vi "tcp client test.vi"() -> ()   [LabVIEW 2015]
panel:
  in  "FUNC":bool
  in  "test":bool=TRUE
  in  "string":string="stastic"
  in  "Direct program":T1
  in  "Boolean":bool
  out "error constant 2":errorcluster
  in  "data":string
  in  "stop":bool
  out "remote address":string
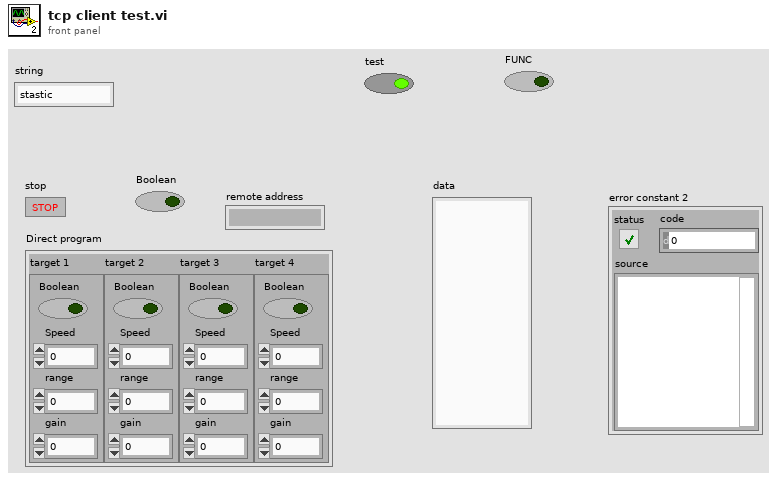
[diagram p1: front panel]
types:
  T1 = cluster{"target 1":cluster{"Boolean":bool, "Speed":dbl, "range":dbl, "gain":dbl}, "target 2":cluster{"Boolean":bool, "Speed":dbl, "range":dbl, "gain":dbl}, "target 3":cluster{"Boolean":bool, "Speed":dbl, "range":dbl, "gain":dbl}, "target 4":cluster{"Boolean":bool, "Speed":dbl, "range":dbl, "gain":dbl}}
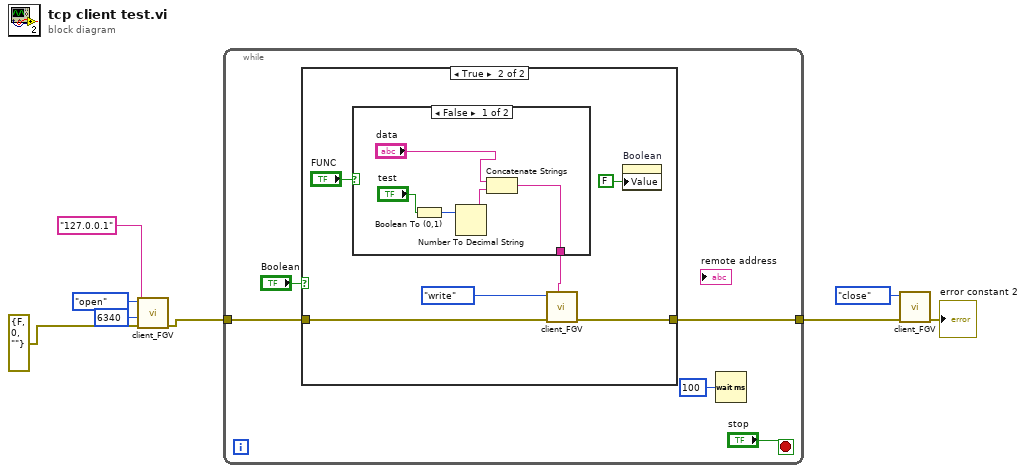
[diagram p0: block diagram]
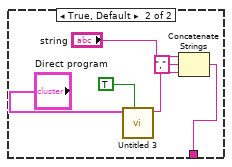
[diagram p3: hidden frame]
diagram:
  n1 = call "client_FGV.vi"("error constant"=errorcluster {"status"=FALSE, "code"=0, "source"=""}, "port"=u16 6340, "address"="127.0.0.1", "Enum"=enum16{"open", "idle", "write", "read", "close"}."open") -> ("error constant 2"=w7:errorcluster)  [unwired: 6 in, 1 out]
  n2 = while {
    tunnel: w7 -> [w11]
    tunnel: [w10] -> w6
    stop <- "stop" stop-if-true
    n3 = case shown="True" "Boolean" {
      tunnel: w11 -> [w14 w20]
      tunnel: [w14 w19] -> w10
      frame False {
      }
      frame True {
        n4 = case shown="False" "FUNC" {
          tunnel: [w25 w29] -> w16
          frame False {
            n5 = Boolean To (0,1)(Boolean="test") -> (0, 1=w23:i16)
            n6 = Number To Decimal String(number=w23) -> (decimal integer string=w22:string)  [unwired: 1 in]
            n7 = Concatenate Strings("data", w22) -> (w25:string)
          }
          frame True, Default {
            n8 = call "Untitled 3.vi"("Boolean"=TRUE, "Direct program"="Direct program") -> ("concatenated string"=w28:string)  [unwired: 8 in, 1 out]
            n9 = Concatenate Strings("string", "," ("string"), w28) -> (w29:string)
          }
        }
        n10 = call "client_FGV.vi"("data in"=w16, "error constant"=w20, "Enum"=enum16{"open", "idle", "write", "read", "close"}."write") -> ("error constant 2"=w19:errorcluster)  [unwired: 7 in, 1 out]
        n11 = property on="Boolean" class="Bool (strict)"("Value"=FALSE ("Boolean")) -> ()  [unwired: 2 in, 2 out]
      }
    }
    n12 = Wait (ms)(milliseconds to wait=u32 100) -> ()  [unwired: 1 out]
  }
  n13 = call "client_FGV.vi"("error constant"=w6, "Enum"=enum16{"open", "idle", "write", "read", "close"}."close") -> ("error constant 2"=→"error constant 2":errorcluster)  [unwired: 8 in, 1 out]
